vi "NV40_Device.vi"(7 "Device-specific in":variant, 8 "error in (no error)":errorcluster, 10 "Position in":dbl[](array[numeric]), 11 "Operation":T2(ring)) -> (0 "error out":errorcluster, 1 "Device properties":cluster{"Axes":string[], "Tolerance":dbl[][]}, 2 "Position out":dbl[](array[numeric]), 3 "Status":T1, 5 "Device-specific out":variant)   [LabVIEW 2015]
uses:
  <vilib>/Instr/_visa.llb/VISA Open Access Mode.ctl
  <vilib>/Instr/_visa.llb/VISA Configure Serial Port (Instr).vi
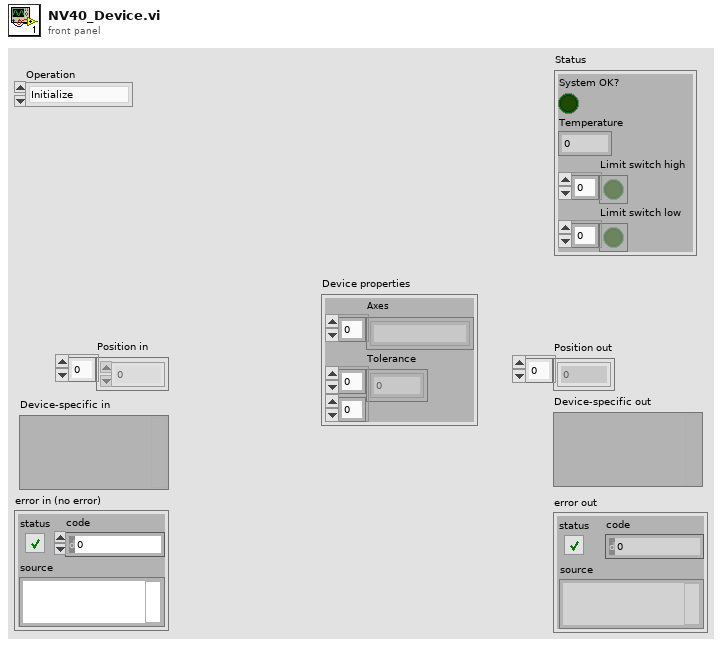
[diagram p1: front panel]
types:
  T1 = cluster{"System OK?":bool, "Temperature":dbl, "Limit switch high":bool[], "Limit switch low":bool[]}
  T2 = enum16{"Initialize", "Shut down", "Set position", "Get position", "Get status", "Other settings"}
  T3 = cluster{"COM port":refnum<visa-resource-name>, "Timeout":u32}
  T4 = typedef "VISA Open Access Mode.ctl" = u32
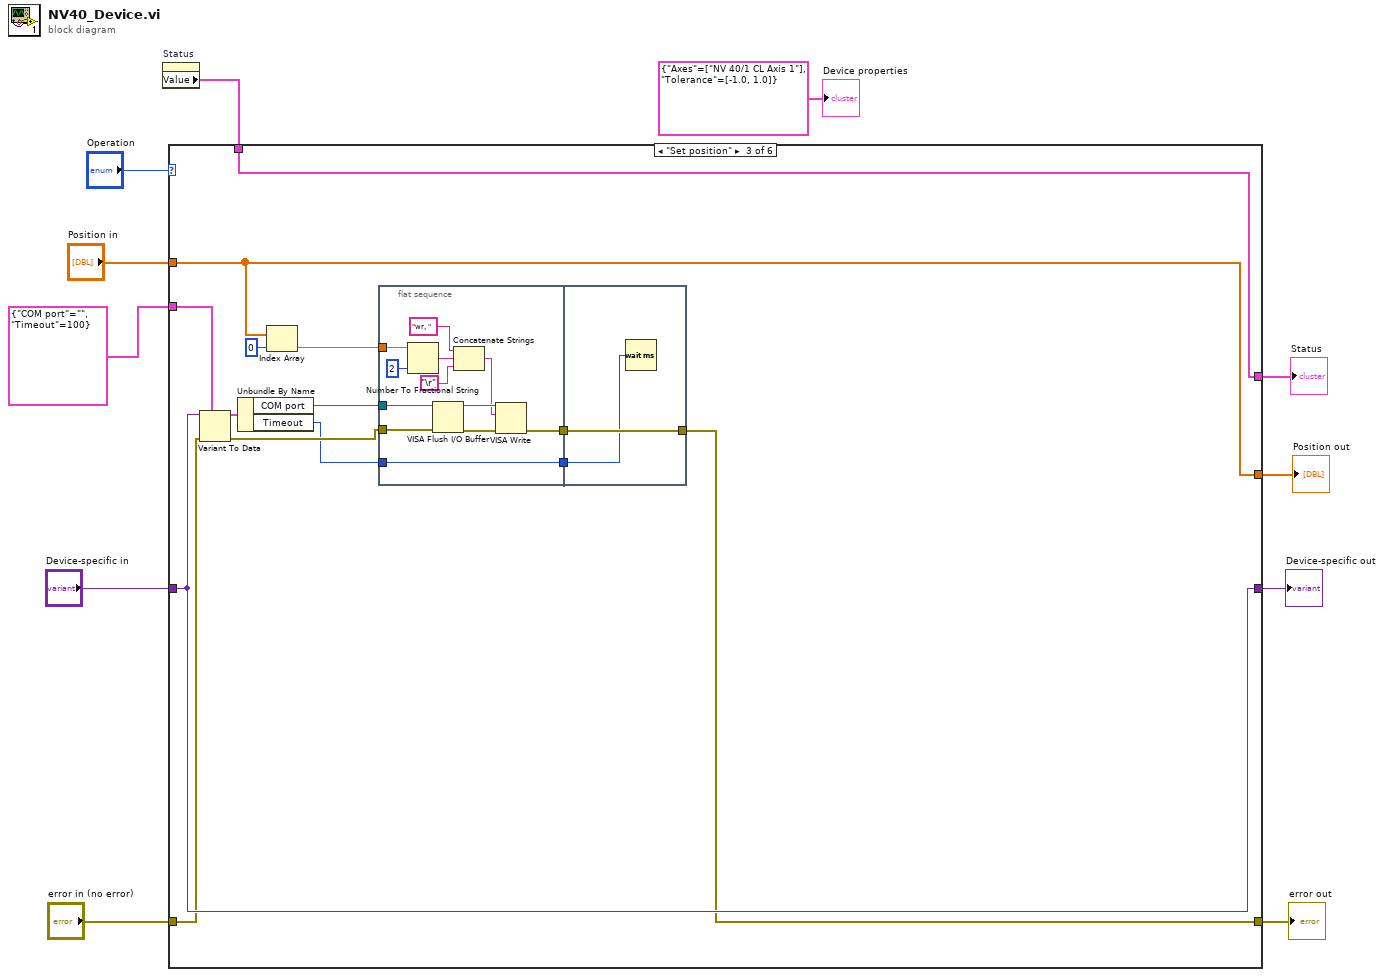
[diagram p0: block diagram]
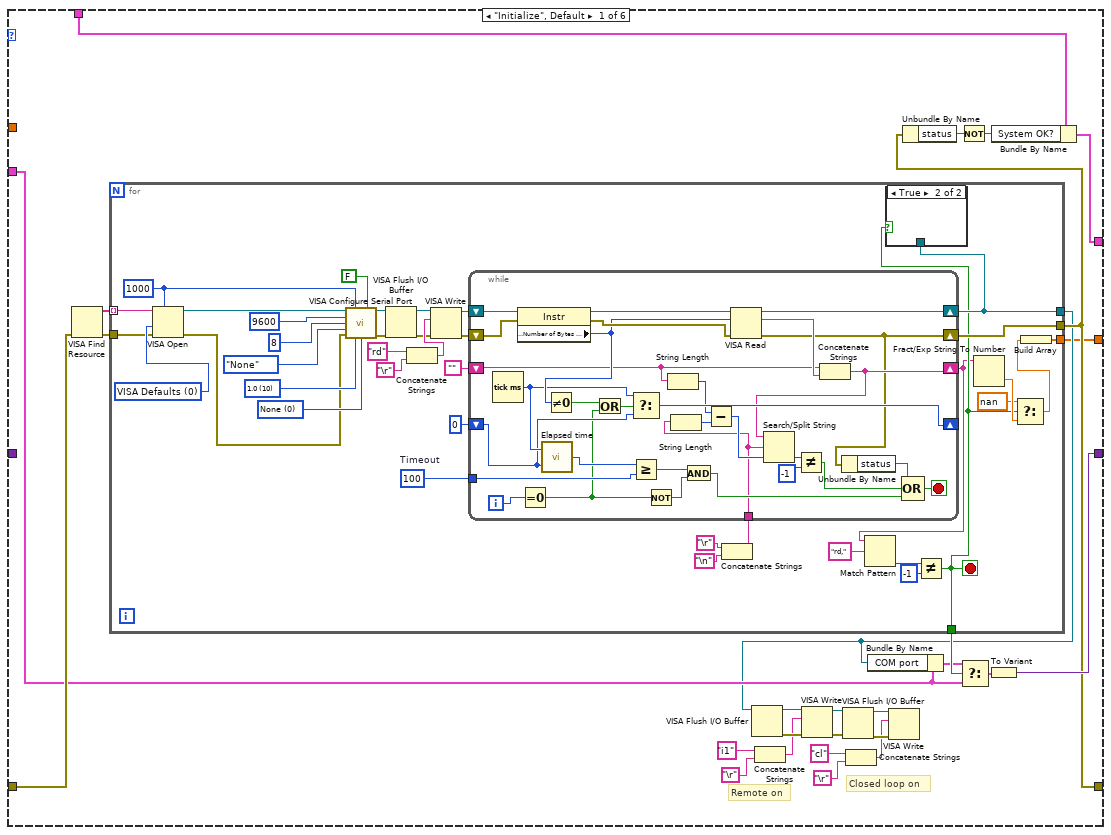
[diagram p2: hidden frame]
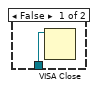
[diagram p3: hidden frame]
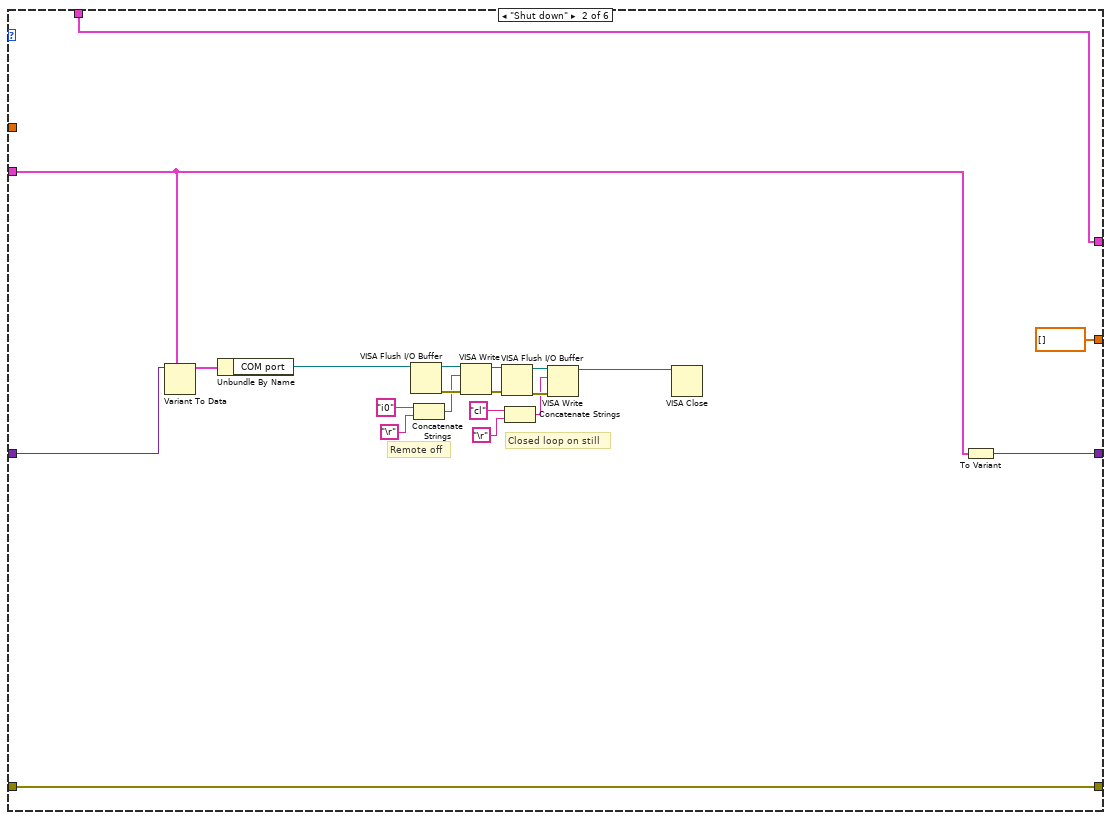
[diagram p4: hidden frame]
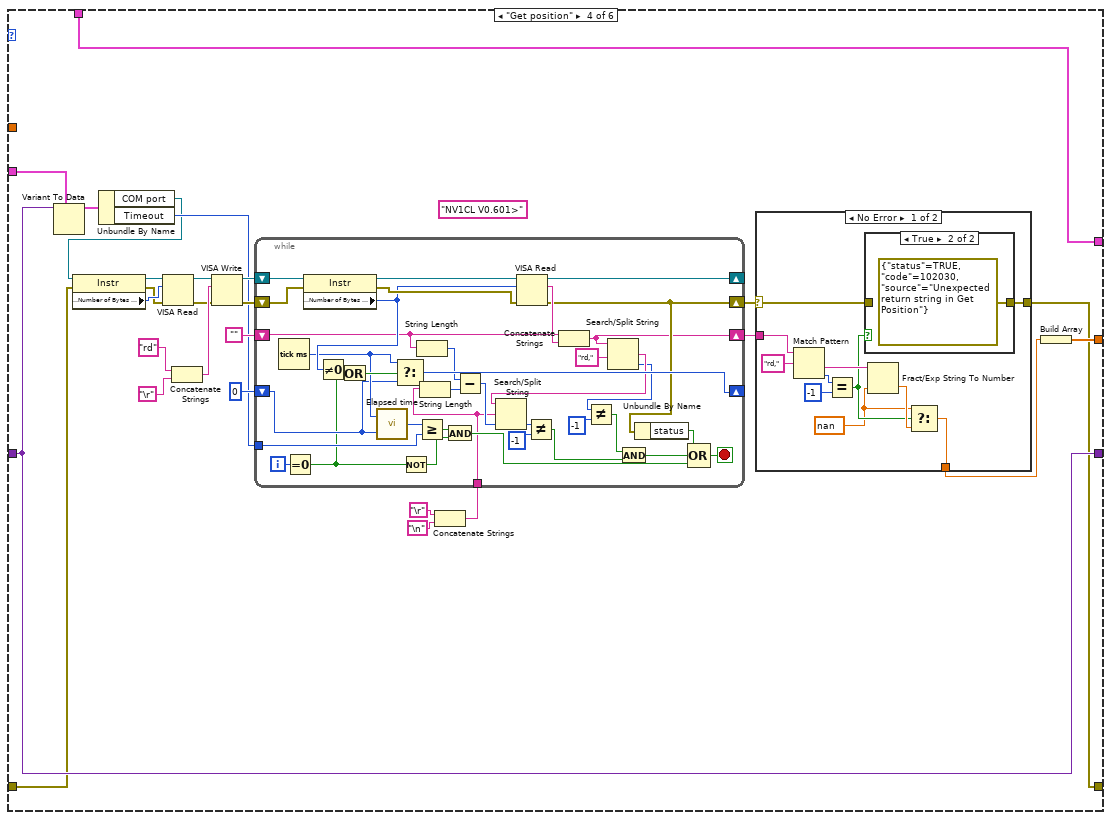
[diagram p5: hidden frame]
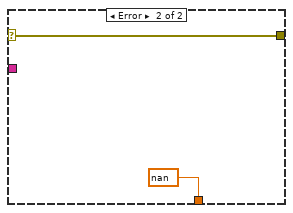
[diagram p7: hidden frame]
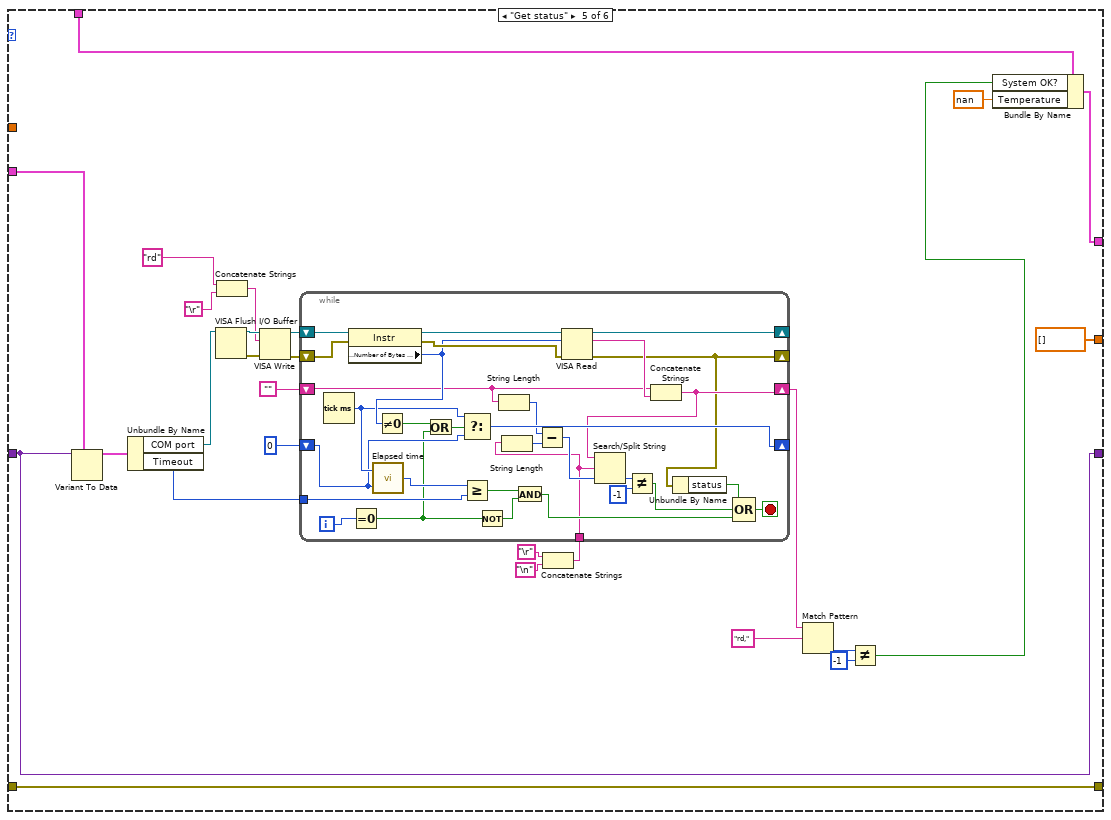
[diagram p8: hidden frame]
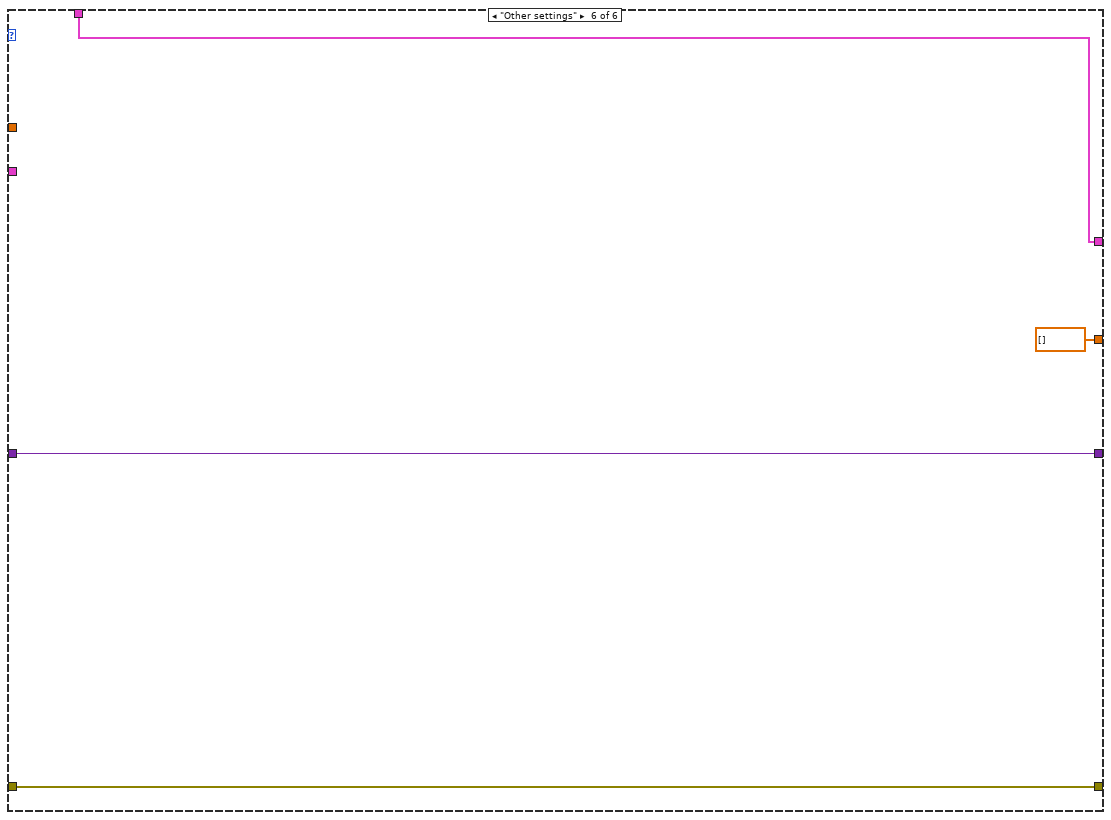
[diagram p9: hidden frame]
diagram:
  n1 = property on="Status" class="Clust (strict)"() -> ("Value"=w10:T1)  [unwired: 2 in, 2 out]
  n2 = case shown="\"Set position\"" "Operation" {
    tunnel: "Position in" -> [_ _ w138 _ _ _]
    tunnel: w10 -> [w38 w129 w143 w184 w263 w298]
    tunnel: [w37 w129 w143 w184 w262 w298] -> w9
    tunnel: "Device-specific in" -> [_ w126 w142 w173 w247 w297]
    tunnel: [w12 dbl[] [] ("Position in") w138 w174 dbl[] [] ("Position in") dbl[] [] ("Position in")] -> w6
    tunnel: [w32 w123 w142 w173 w247 w297] -> w5
    tunnel: [w29 w128 w133 w166 w260 w296] -> w4
    tunnel: "error in (no error)" -> [w30 w128 w134 w161 w260 w296]
    tunnel: T3 {"COM port"="", "Timeout"=100} -> [w27 w124 w141 w172 w246 _]
    frame "Initialize", Default {
      # "Remote on"
      # "Closed loop on"
      n3 = VISA Find Resource(8:w30) -> (0:w31:errorcluster, 3:w36:string[])  [unwired: 2 in, 1 out]
      n4 = for {
        tunnel: w36 -> [w66] mode=indexing
        tunnel: [w46] -> w13
        tunnel: [w42] -> w35
        tunnel: w31 -> [w48]
        tunnel: [w47] -> w29
        tunnel: [w39] -> w12
        stop <- w42 stop-if-true
        w56 = u32 100  # Timeout
        w67 = u32 1000 ("timeout (10sec)")
        w69 = T4 0 items=["VISA Defaults"=0, "Exclusive Lock"=1, "Load Configured Settings"=4] ("Access Mode")
        w71 = u16 0 items=["None", "XON/XOFF", "RTS/CTS", "XON/XOFF & RTS/CTS", "DTR/DSR", "XON/XOFF & DTR/DSR"] ("flow control (0:none)")
        w72 = u16 10 items=["1.0"=10, "1.5"=15, "2.0"=20] ("stop bits (10: 1 bit)")
        n5 = VISA Open(timeout (0)=w67, access mode=w69, error in (no error)=w48, VISA resource name=w66) -> (VISA resource name=w70:refnum<visa-resource-name>, error out=w68:errorcluster)  [unwired: 1 in]
        n6 = call-poly "VISA Configure Serial Port"("VISA resource name"=w70, "timeout (10sec)"=w67, "Enable Termination\nChar (T)"=FALSE ("Enable Termination\nChar (T)"), "baud rate (9600)"=u32 9600, "data bits (8)"=u16 8, "parity (0:none)"=enum16{"None", "Odd", "Even", "Mark", "Space"}."None", "error in (no error)"=w68, "stop bits (10: 1 bit)"=w72, "flow control (0:none)"=w71) -> ("VISA resource name out"=w51:refnum<visa-resource-name>, "error out"=w52:errorcluster)  [unwired: 5 in]
        n7 = VISA Flush I/O Buffer(VISA resource name=w51, error in (no error)=w52) -> (VISA resource name out=w64:refnum<visa-resource-name>, error out=w62:errorcluster)  [unwired: 1 in]
        n8 = Concatenate Strings("rd", "\r") -> (w63:string)
        n9 = VISA Write(VISA resource name=w64, write buffer=w63, error in (no error)=w62) -> (VISA resource name out=w61:refnum<visa-resource-name>, error out=w60:errorcluster)  [unwired: 1 out]
        n10 = Concatenate Strings("\r", "\n") -> (w53:string)
        n11 = while {
          shift-right: [w104] -> w46
          shift-left: w61 -> [w108]
          shift-right: [w78] -> w47
          shift-left: w60 -> [w107]
          shift-right: [w85] -> w41
          shift-left: "" -> [w84]
          shift-right: [w93] -> _
          shift-left: u32 0 -> [w90]
          tunnel: w56 -> [w91]
          tunnel: w53 -> [w79]
          i -> [w96]
          stop <- w103 stop-if-true
          n12 = Tick Count (ms)() -> (millisecond timer value=w94:u32)
          n13 = property class="Instr"(reference=w108, error in=w107) -> (reference out=w106:refnum<visa-resource-name>, error out=w105:errorcluster, "Serial Settings:Number of Bytes at Serial Port"=w98:u32)
          n14 = Equal To 0?(x=w96) -> (x = 0?=w86:bool)
          n15 = call "Elapsed time.vi"("Start time (ms)"=w90, "Current time (ms)"=w94) -> ("Elapsed time"=w92:u32)
          n16 = Not Equal To 0?(x=w98) -> (x != 0?=w97:bool)
          n17 = Or(x=w97, y=w86) -> (x .or. y?=w95:bool)
          n18 = Select(t=w94, s=w95, f=w90) -> (s? t:f=w93:u32)
          n19 = Greater Or Equal?(x=w92, y=w91) -> (x >= y?=w88:bool)
          n20 = Not(x=w86) -> (.not. x?=w87:bool)
          n21 = String Length(string=w84) -> (length=w82:i32)
          n22 = String Length(string=w79) -> (length=w83:i32)
          n23 = And(x=w88, y=w87) -> (x .and. y?=w89:bool)
          n24 = Subtract(x=w82, y=w83) -> (x-y=w81:i32)
          n25 = VISA Read(VISA resource name=w106, byte count=w98, error in (no error)=w105) -> (VISA resource name out=w104:refnum<visa-resource-name>, read buffer=w102:string, error out=w78:errorcluster)  [unwired: 1 out]
          n26 = Concatenate Strings(w84, w102) -> (w85:string)
          n27 = Search/Split String(string=w85, search string/char (-)=w79, offset (0)=w81) -> (offset of match=w101:i32)  [unwired: 2 out]
          n28 = Not Equal?(x=w101, y=-1) -> (x != y?=w99:bool)
          n29 = Unbundle By Name(w78) -> ("status"=w80:bool)
          n30 = Compound Arithmetic op=OR(w80, w99, w89) -> (w103:bool)
        }
        n31 = Match Pattern(string=w41, regular expression="rd,") -> (offset past match=w50:i32)  [unwired: 1 in, 3 out]
        n32 = Not Equal?(x=w50, y=-1) -> (x != y?=w42:bool)
        n33 = case shown="True" w42 {
          tunnel: w46 -> [w77 _]
          frame False {
            n34 = VISA Close(VISA resource name=w77) -> ()  [unwired: 1 in, 1 out]
          }
          frame True {
          }
        }
        n35 = Fract/Exp String To Number(string=w41) -> (number=w44:dbl)  [unwired: 3 in, 1 out]
        n36 = Select(t=nan, s=w42, f=w44) -> (s? t:f=w40:dbl)
        n37 = Build Array(w40) -> (w39:dbl[])
      }
      n38 = VISA Flush I/O Buffer(VISA resource name=w13) -> (VISA resource name out=w25:refnum<visa-resource-name>, error out=w24:errorcluster)  [unwired: 2 in]
      n39 = Concatenate Strings("i1" ("string"), "\r") -> (w23:string)
      n40 = VISA Write(VISA resource name=w25, write buffer=w23, error in (no error)=w24) -> (VISA resource name out=w15:refnum<visa-resource-name>, error out=w14:errorcluster)  [unwired: 1 out]
      n41 = VISA Flush I/O Buffer(VISA resource name=w15, error in (no error)=w14) -> (VISA resource name out=w20:refnum<visa-resource-name>, error out=w19:errorcluster)  [unwired: 1 in]
      n42 = Concatenate Strings("cl" ("string"), "\r") -> (w18:string)
      n43 = Bundle By Name(cluster=w27, "COM port"=w13) -> (w34:T3)
      n44 = VISA Write(VISA resource name=w20, write buffer=w18, error in (no error)=w19) -> ()  [unwired: 3 out]
      n45 = Unbundle By Name(w29) -> ("status"=w28:bool)
      n46 = Not(x=w28) -> (.not. x?=w26:bool)
      n47 = Select(t=w34, s=w35, f=w27) -> (s? t:f=w33:T3)
      n48 = To Variant(anything=w33) -> (Variant=w32:variant)
      n49 = Bundle By Name(cluster=w38, "System OK?"=w26) -> (w37:T1)
    }
    frame "Shut down" {
      # "Remote off"
      # "Closed loop on still"
      n50 = Variant To Data(type=w124, Variant=w126) -> (data=w125:T3)  [unwired: 1 in, 1 out]
      n51 = Unbundle By Name(w125) -> ("COM port"=w110:refnum<visa-resource-name>)
      n52 = VISA Flush I/O Buffer(VISA resource name=w110) -> (VISA resource name out=w122:refnum<visa-resource-name>, error out=w121:errorcluster)  [unwired: 2 in]
      n53 = Concatenate Strings("i0" ("string"), "\r") -> (w120:string)
      n54 = VISA Write(VISA resource name=w122, write buffer=w120, error in (no error)=w121) -> (VISA resource name out=w112:refnum<visa-resource-name>, error out=w111:errorcluster)  [unwired: 1 out]
      n55 = VISA Flush I/O Buffer(VISA resource name=w112, error in (no error)=w111) -> (VISA resource name out=w117:refnum<visa-resource-name>, error out=w116:errorcluster)  [unwired: 1 in]
      n56 = Concatenate Strings("cl" ("string"), "\r") -> (w115:string)
      n57 = VISA Write(VISA resource name=w117, write buffer=w115, error in (no error)=w116) -> (VISA resource name out=w109:refnum<visa-resource-name>)  [unwired: 2 out]
      n58 = VISA Close(VISA resource name=w109) -> ()  [unwired: 1 in, 1 out]
      n59 = To Variant(anything=w124) -> (Variant=w123:variant)
    }
    frame "Set position" {
      n60 = Variant To Data(error in=w134, type=w141, Variant=w142) -> (data=w140:T3, error out=w135:errorcluster)
      n61 = Unbundle By Name(w140) -> ("COM port"=w139:refnum<visa-resource-name>, "Timeout"=w130:u32)
      n62 = Index Array(array=w138, index=0) -> (element=w137:dbl)
      n63 = flat-sequence {
        tunnel: w139 -> [w153]
        tunnel: w137 -> [w150]
        tunnel: w135 -> [w146]
        tunnel: [w145] -> w132
        tunnel: [w144] -> w131
        tunnel: w130 -> [w144]
        tunnel: [w157] -> w133
        tunnel: w132 -> [w157]
        tunnel: w131 -> [w156]
        frame #0 {
          n64 = Number To Fractional String(number=w150, precision (6)=i16 2) -> (F-format string=w151:string)  [unwired: 2 in]
          n65 = VISA Flush I/O Buffer(VISA resource name=w153, error in (no error)=w146) -> (VISA resource name out=w155:refnum<visa-resource-name>, error out=w154:errorcluster)  [unwired: 1 in]
          n66 = Concatenate Strings("wr, ", w151, "\r") -> (w149:string)
          n67 = VISA Write(VISA resource name=w155, write buffer=w149, error in (no error)=w154) -> (error out=w145:errorcluster)  [unwired: 2 out]
        }
        frame #1 {
          n68 = Wait (ms)(milliseconds to wait=w156) -> ()  [unwired: 1 out]
        }
      }
    }
    frame "Get position" {
      (unwired) "NV1CL V0.601>"
      n69 = Variant To Data(type=w172, Variant=w173) -> (data=w171:T3)  [unwired: 1 in, 1 out]
      n70 = Unbundle By Name(w171) -> ("COM port"=w160:refnum<visa-resource-name>, "Timeout"=w170:u32)
      n71 = property class="Instr"(reference=w160, error in=w161) -> (reference out=w163:refnum<visa-resource-name>, error out=w162:errorcluster, "Serial Settings:Number of Bytes at Serial Port"=w164:u32)
      n72 = VISA Read(VISA resource name=w163, byte count=w164, error in (no error)=w162) -> (VISA resource name out=w159:refnum<visa-resource-name>, error out=w158:errorcluster)  [unwired: 2 out]
      n73 = Concatenate Strings("rd", "\r") -> (w182:string)
      n74 = VISA Write(VISA resource name=w159, write buffer=w182, error in (no error)=w158) -> (VISA resource name out=w181:refnum<visa-resource-name>, error out=w180:errorcluster)  [unwired: 1 out]
      n75 = Concatenate Strings("\r", "\n") -> (w175:string)
      n76 = while {
        shift-right: [w232] -> _
        shift-left: w181 -> [w236]
        shift-right: [w208] -> w168
        shift-left: w180 -> [w235]
        shift-right: [w207] -> w167
        shift-left: "" -> [w214]
        shift-right: [w222] -> _
        shift-left: u32 0 -> [w219]
        tunnel: w170 -> [w220]
        tunnel: w175 -> [w209]
        i -> [w225]
        stop <- w231 stop-if-true
        n77 = Tick Count (ms)() -> (millisecond timer value=w223:u32)
        n78 = Equal To 0?(x=w225) -> (x = 0?=w215:bool)
        n79 = property class="Instr"(reference=w236, error in=w235) -> (reference out=w234:refnum<visa-resource-name>, error out=w233:errorcluster, "Serial Settings:Number of Bytes at Serial Port"=w227:u32)
        n80 = Not Equal To 0?(x=w227) -> (x != 0?=w226:bool)
        n81 = Or(x=w226, y=w215) -> (x .or. y?=w224:bool)
        n82 = call "Elapsed time.vi"("Start time (ms)"=w219, "Current time (ms)"=w223) -> ("Elapsed time"=w221:u32)
        n83 = Select(t=w223, s=w224, f=w219) -> (s? t:f=w222:u32)
        n84 = Not(x=w215) -> (.not. x?=w216:bool)
        n85 = String Length(string=w214) -> (length=w212:i32)
        n86 = Greater Or Equal?(x=w221, y=w220) -> (x >= y?=w217:bool)
        n87 = String Length(string=w209) -> (length=w213:i32)
        n88 = And(x=w217, y=w216) -> (x .and. y?=w218:bool)
        n89 = Subtract(x=w212, y=w213) -> (x-y=w211:i32)
        n90 = VISA Read(VISA resource name=w234, byte count=w227, error in (no error)=w233) -> (VISA resource name out=w232:refnum<visa-resource-name>, read buffer=w230:string, error out=w208:errorcluster)  [unwired: 1 out]
        n91 = Concatenate Strings(w214, w230) -> (w207:string)
        n92 = Search/Split String(string=w207, search string/char (-)="rd,") -> (match + rest of string=w205:string, offset of match=w203:i32)  [unwired: 1 in, 1 out]
        n93 = Search/Split String(string=w205, search string/char (-)=w209, offset (0)=w211) -> (offset of match=w229:i32)  [unwired: 2 out]
        n94 = Not Equal?(x=w229, y=-1) -> (x != y?=w202:bool)
        n95 = Not Equal?(x=w203, y=-1) -> (x != y?=w201:bool)
        n96 = And(x=w201, y=w202) -> (x .and. y?=w200:bool)
        n97 = Unbundle By Name(w208) -> ("status"=w210:bool)
        n98 = Compound Arithmetic op=OR(w210, w200, w218) -> (w231:bool)
      }
      n99 = case shown="No Error" w168 {
        selector: w168 -> [w189 w199]
        tunnel: w167 -> [w195 _]
        tunnel: [w190 w199] -> w166
        tunnel: [w188 nan] -> w165
        frame No Error {
          w185 = nan ("t")
          n100 = Match Pattern(string=w195, regular expression="rd,") -> (after substring=w193:string, offset past match=w192:i32)  [unwired: 1 in, 2 out]
          n101 = Equal?(x=w192, y=-1) -> (x = y?=w186:bool)
          n102 = case shown="True" w186 {
            tunnel: [w196 errorcluster {"status"=TRUE, "code"=102030, "source"="Unexpected return string in Get Position"} ("error IO")] -> w190
            tunnel: w189 -> [w196 _]
            frame False {
            }
            frame True {
            }
          }
          n103 = Fract/Exp String To Number(string=w193, default (0 dbl)=w185) -> (number=w187:dbl)  [unwired: 2 in, 1 out]
          n104 = Select(t=w185, s=w186, f=w187) -> (s? t:f=w188:dbl)
        }
        frame Error {
        }
      }
      n105 = Build Array(w165) -> (w174:dbl[])
    }
    frame "Get status" {
      n106 = Variant To Data(type=w246, Variant=w247) -> (data=w245:T3)  [unwired: 1 in, 1 out]
      n107 = Unbundle By Name(w245) -> ("COM port"=w243:refnum<visa-resource-name>, "Timeout"=w244:u32)
      n108 = VISA Flush I/O Buffer(VISA resource name=w243) -> (VISA resource name out=w258:refnum<visa-resource-name>, error out=w257:errorcluster)  [unwired: 2 in]
      n109 = Concatenate Strings("rd", "\r") -> (w248:string)
      n110 = VISA Write(VISA resource name=w258, write buffer=w248, error in (no error)=w257) -> (VISA resource name out=w256:refnum<visa-resource-name>, error out=w255:errorcluster)  [unwired: 1 out]
      n111 = Concatenate Strings("\r", "\n") -> (w250:string)
      n112 = while {
        shift-right: [w290] -> _
        shift-left: w256 -> [w294]
        shift-right: [w264] -> _
        shift-left: w255 -> [w293]
        shift-right: [w271] -> w242
        shift-left: "" -> [w270]
        shift-right: [w279] -> _
        shift-left: u32 0 -> [w276]
        tunnel: w244 -> [w277]
        tunnel: w250 -> [w265]
        i -> [w282]
        stop <- w289 stop-if-true
        n113 = Tick Count (ms)() -> (millisecond timer value=w280:u32)
        n114 = property class="Instr"(reference=w294, error in=w293) -> (reference out=w292:refnum<visa-resource-name>, error out=w291:errorcluster, "Serial Settings:Number of Bytes at Serial Port"=w284:u32)
        n115 = Equal To 0?(x=w282) -> (x = 0?=w272:bool)
        n116 = call "Elapsed time.vi"("Start time (ms)"=w276, "Current time (ms)"=w280) -> ("Elapsed time"=w278:u32)
        n117 = Not Equal To 0?(x=w284) -> (x != 0?=w283:bool)
        n118 = Or(x=w283, y=w272) -> (x .or. y?=w281:bool)
        n119 = Select(t=w280, s=w281, f=w276) -> (s? t:f=w279:u32)
        n120 = Greater Or Equal?(x=w278, y=w277) -> (x >= y?=w274:bool)
        n121 = Not(x=w272) -> (.not. x?=w273:bool)
        n122 = String Length(string=w270) -> (length=w268:i32)
        n123 = String Length(string=w265) -> (length=w269:i32)
        n124 = And(x=w274, y=w273) -> (x .and. y?=w275:bool)
        n125 = Subtract(x=w268, y=w269) -> (x-y=w267:i32)
        n126 = VISA Read(VISA resource name=w292, byte count=w284, error in (no error)=w291) -> (VISA resource name out=w290:refnum<visa-resource-name>, read buffer=w288:string, error out=w264:errorcluster)  [unwired: 1 out]
        n127 = Concatenate Strings(w270, w288) -> (w271:string)
        n128 = Search/Split String(string=w271, search string/char (-)=w265, offset (0)=w267) -> (offset of match=w287:i32)  [unwired: 2 out]
        n129 = Not Equal?(x=w287, y=-1) -> (x != y?=w285:bool)
        n130 = Unbundle By Name(w264) -> ("status"=w266:bool)
        n131 = Compound Arithmetic op=OR(w266, w285, w275) -> (w289:bool)
      }
      n132 = Match Pattern(string=w242, regular expression="rd,") -> (offset past match=w240:i32)  [unwired: 1 in, 3 out]
      n133 = Not Equal?(x=w240, y=-1) -> (x != y?=w238:bool)
      n134 = Bundle By Name(cluster=w263, "System OK?"=w238, "Temperature"=nan) -> (w262:T1)
    }
    frame "Other settings" {
    }
  }
  "Status" <- w9
  "Device-specific out" <- w5
  "error out" <- w4
  "Position out" <- w6
  "Device properties" <- cluster{"Axes":string[], "Tolerance":dbl[][]} {"Axes"=["NV 40/1 CL Axis 1"], "Tolerance"=[[-1.0, 1.0]]} ("Device properties")
